vi "CRYSet Probe Result Front Panel.vi"(11 "Vi Ref":refnum<vi>) -> ()   [LabVIEW 2013]
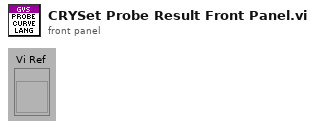
[diagram p1: front panel]
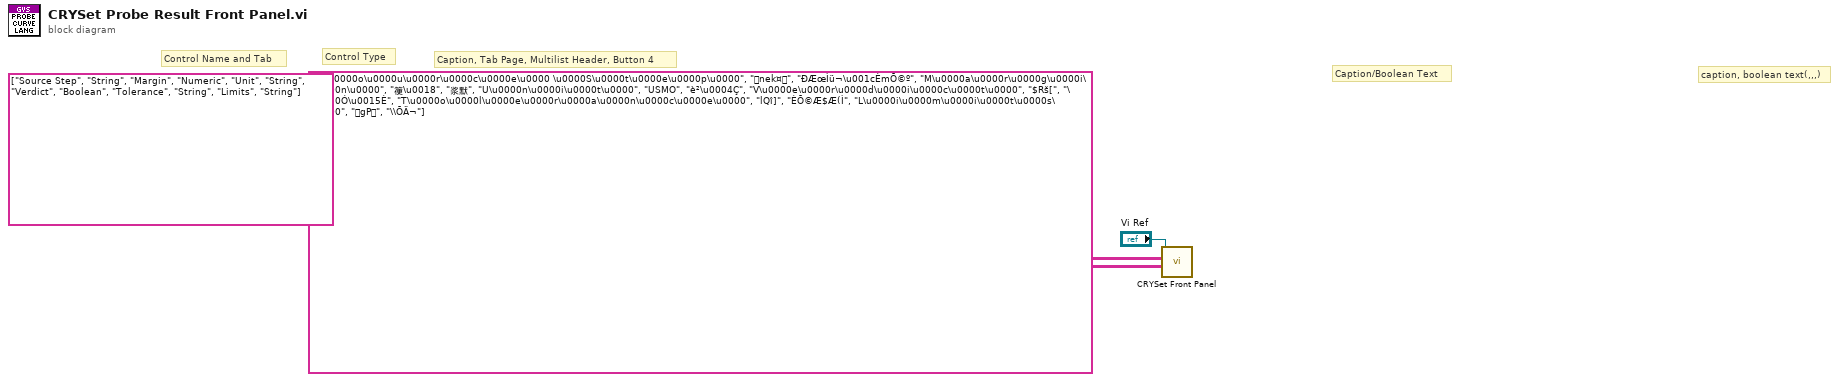
[diagram p0: block diagram]
diagram:
  # "Caption, Tab Page, Multilist Header, Button 4"
  # "Control Type"
  # "Control Name and Tab"
  # "caption, boolean text(,,,)"
  # "Caption/Boolean Text"
  n1 = call "CRYSet Front Panel.vi"("Caption(Boolean Text)"=string[][] [["S\u0000o\u0000u\u0000r\u0000c\u0000e\u0000 \u0000S\u0000t\u0000e\u0000p\u0000", "nek¤", "ÐÆœÌü¬\u001cÈmÕ©º"], ["M\u0000a\u0000r\u0000g\u0000i\u0000n\u0000", "箯\u0018", "浆默"], ["U\u0000n\u0000i\u0000t\u0000", "USMO", "è²\u0004Ç"], ["V\u0000e\u0000r\u0000d\u0000i\u0000c\u0000t\u0000", "$Rš[", "\u0010Ó\u0015È"], ["T\u0000o\u0000l\u0000e\u0000r\u0000a\u0000n\u0000c\u0000e\u0000", "lQî]", "ÈÕ©Æ$Æ(Ì"], ["L\u0000i\u0000m\u0000i\u0000t\u0000s\u0000", "gP", "\\ÕÄ¬"]], "Control ID and Type(Label Name, Type)"=string[][] [["Source Step", "String"], ["Margin", "Numeric"], ["Unit", "String"], ["Verdict", "Boolean"], ["Tolerance", "String"], ["Limits", "String"]], "Vi Ref"="Vi Ref") -> ()  [unwired: 9 in]
